vi "Handle Dirty Elements.vi"(8 "Update Time":i32=100, 10 "notifier out":refnum<notifier>, 11 "IsClient":bool) -> (2 "notifier out 2":refnum<notifier>)   [LabVIEW 2017]
doc: "Based on the update rate of this client, keep track of elements that are dirty - have been written to locally. Propagate those values to other clients. This VI also injects statistical measurements of the NT traffic and stores modified value to the persistence file if the variable has been marked as persistent."
uses:
  <vilib>/Rock Robotics/Network Tables/Make Table Operation.ctl
  <vilib>/Rock Robotics/Network Tables/NT Globals.vi
panel:
  in  "Usage Report Period":dbl=0.5
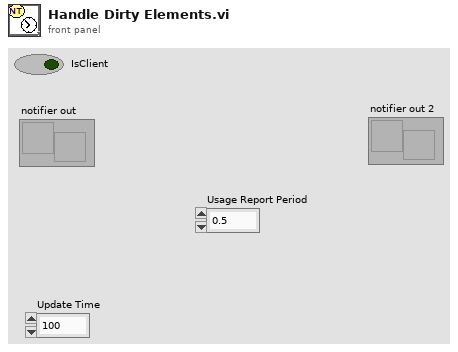
[diagram p1: front panel]
types:
  T1 = enum16{"Add Cnx", "Remove Cnx", "Retrieve List", "Cnx Inited"}
  T2 = typedef "Make Table Operation.ctl" = enum16{"Get or Add Field", "Get Field or Add Temp", "Replace Temp ID", "Get Field ID - No Add", "Get Table Field IDs", "Get Field ID Info", "Move Field to Temp", "Validate", "Remove Field", "Remove All"}
  T3 = typedef "Field ID.ctl" = i32
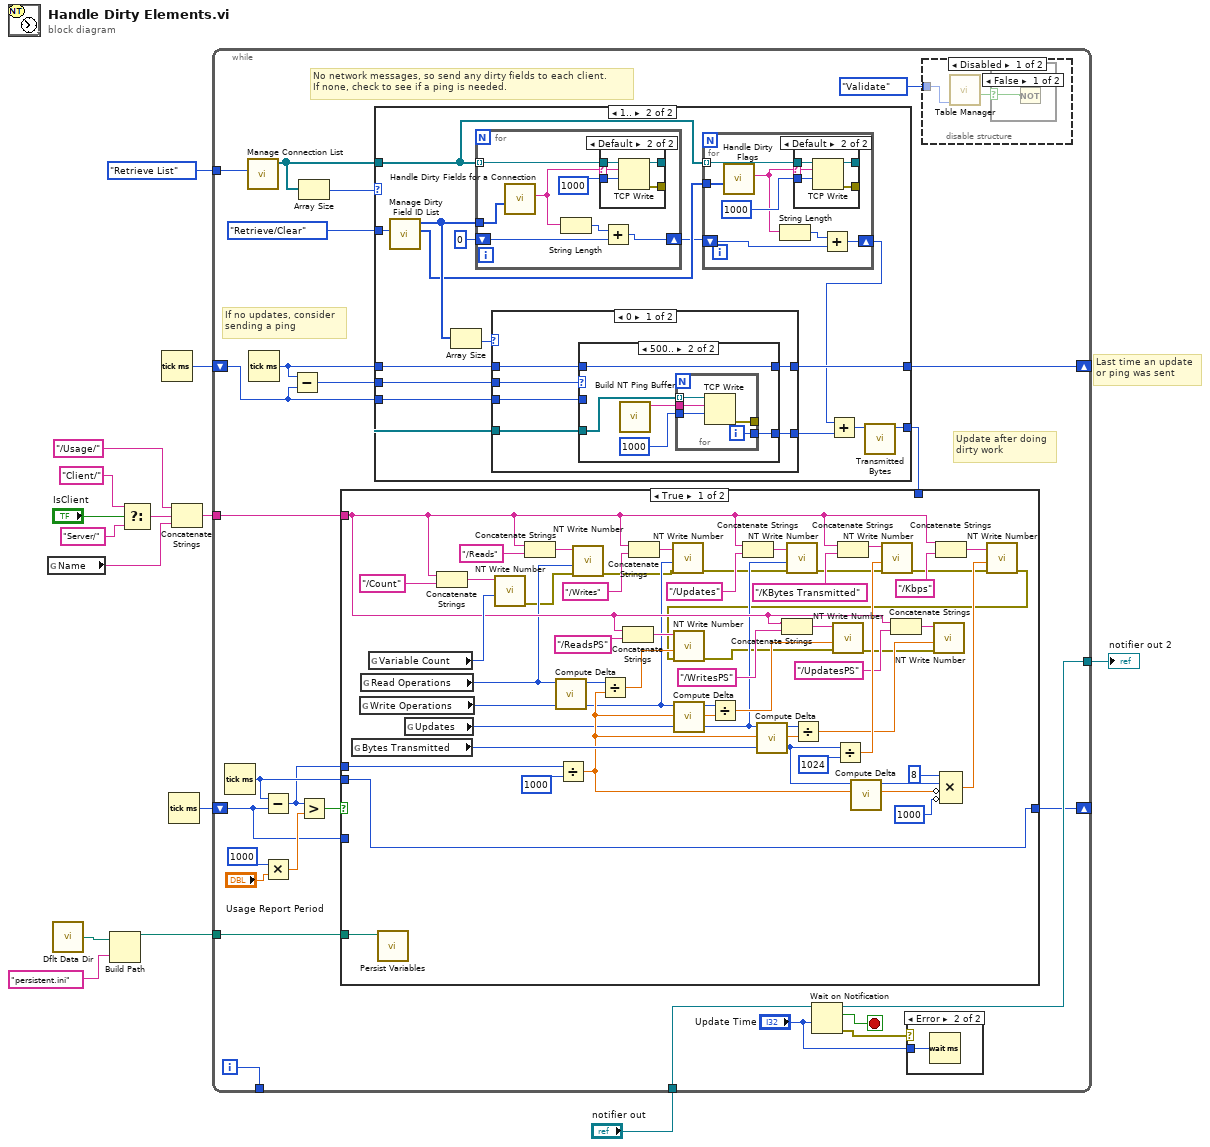
[diagram p0: block diagram]
diagram:
  # "Last time an update\nor ping was sent"
  n1 = global read "NT Globals.vi" "Name"() -> (w12:string)
  n2 = call <vilib>:"Dflt Data Dir.vi"() -> ("App:Default Data Directory"=w1:path)
  n3 = Build Path(base path=w1, name or relative path="persistent.ini") -> (appended path=w2:path)
  n4 = Select(t="Client/" ("Name"), s="IsClient", f="Server/" ("Name")) -> (s? t:f=w11:string)
  n5 = Tick Count (ms)() -> (millisecond timer value=w15:u32)
  n6 = Tick Count (ms)() -> (millisecond timer value=w5:u32)
  n7 = Concatenate Strings("/Usage/" ("Name"), w11, w12) -> (w7:string)
  n8 = while {
    shift-right: [w40] -> _
    shift-left: w15 -> [w34]
    tunnel: "notifier out" -> [w39]
    tunnel: [w38] -> w13
    tunnel: w7 -> [w36]
    tunnel: [w32] -> _
    shift-right: [w26] -> _
    shift-left: w5 -> [w24]
    tunnel: T1."Retrieve List" ("Operation") -> [w17]
    tunnel: w2 -> [w16]
    i -> [w32]
    stop <- w37 stop-if-true
    # "Update after doing\ndirty work"
    # "No network messages, so send any dirty fields to each client.\nIf none, check to see if a ping is needed."
    # "If no updates, consider\nsending a ping"
    n9 = Tick Count (ms)() -> (millisecond timer value=w25:u32)
    n10 = call <vilib>:"Manage Connection List.vi"("Operation"=w17) -> ("Connections List"=w21:refnum<k5>[])  [unwired: 8 in, 2 out]
    n11 = Tick Count (ms)() -> (millisecond timer value=w35:u32)
    n12 = Subtract(x=w25, y=w24) -> (x-y=w23:u32)
    n13 = Multiply(x=1000, y="Usage Report Period") -> (x*y=w27:dbl)
    n14 = Subtract(x=w35, y=w34) -> (x-y=w33:u32)
    n15 = Array Size(array=w21) -> (size(s)=w20:i32)
    n16 = Greater?(x=w23, y=w27) -> (0:w18:bool)
    n17 = case shown="1.." w20 {
      tunnel: enum16{"Mark", "Retrieve/Clear"}."Retrieve/Clear" ("Operation") -> [_ w60]
      tunnel: [w45 w59] -> w40
      tunnel: w35 -> [_ w55]
      tunnel: w34 -> [w45 w54]
      tunnel: w33 -> [_ w53]
      tunnel: w21 -> [_ w48]
      tunnel: [_ w50] -> w19
      frame 0, Default {
      }
      frame 1.. {
        n18 = call <vilib>:"Manage Dirty Field ID List.vi"("Operation"=w60) -> ("Field IDs Flags"=w49:T3[], "Field IDs"=w52:T3[])  [unwired: 9 in]
        n19 = Array Size(array=w52) -> (size(s)=w58:i32)
        n20 = for {
          tunnel: w48 -> [w98] mode=indexing
          tunnel: w52 -> [w97]
          shift-right: [w92] -> w47
          shift-left: 0 -> [w93]
          n21 = call <vilib>:"Handle Dirty Fields for a Connection.vi"("Field IDs"=w97) -> ("String out"=w94:string)  [unwired: 10 in]
          n22 = String Length(string=w94) -> (length=w95:i32)
          n23 = case shown="Default" w94 {
            selector: w94 -> [_ w101]
            tunnel: [_ w104] -> _
            tunnel: [w99 w103] -> _
            tunnel: w98 -> [w99 w102]
            tunnel: 1000 ("timeout ms (25000)") -> [_ w100]
            frame "" {
            }
            frame Default {
              n24 = TCP Write(connection ID=w102, data in=w101, 9:w100) -> (connection ID out=w103:refnum<k5>, error out=w104:errorcluster)  [unwired: 1 in, 1 out]
            }
          }
          n25 = Add(x=w95, y=w93) -> (x+y=w92:i32)
        }
        n26 = case shown="0" w58 {
          tunnel: [w78 w91] -> w59
          tunnel: w55 -> [w79 w91]
          tunnel: w54 -> [w77 _]
          tunnel: w48 -> [w76 _]
          tunnel: [w75 _] -> w57
          tunnel: w53 -> [w74 _]
          frame 0 {
            n27 = case shown="500.." w74 {
              tunnel: w79 -> [_ w85]
              tunnel: [w80 w85] -> w78
              tunnel: w77 -> [w80 _]
              tunnel: w76 -> [_ w83]
              tunnel: [_ w82] -> w75
              frame 0, Default {
              }
              frame 500.. {
                n28 = call <vilib>:"Build NT Ping Buffer.vi"() -> ("Data Buffer"=w84:string)  [unwired: 11 in]
                n29 = for {
                  tunnel: w84 -> [w89]
                  tunnel: w83 -> [w90] mode=indexing
                  tunnel: [w88] -> _
                  tunnel: [w87] -> w82
                  tunnel: 1000 ("timeout ms (25000)") -> [w86]
                  i -> [w87]
                  n30 = TCP Write(connection ID=w90, data in=w89, 9:w86) -> (error out=w88:errorcluster)  [unwired: 1 in, 2 out]
                }
              }
            }
          }
          frame 1, Default {
          }
        }
        n31 = for {
          tunnel: w49 -> [w67]
          tunnel: w48 -> [w65] mode=indexing
          shift-right: [w62] -> w46
          shift-left: w47 -> [w63]
          n32 = call <vilib>:"Handle Dirty Flags.vi"("Field IDs"=w67) -> ("String out"=w61:string)  [unwired: 10 in]
          n33 = String Length(string=w61) -> (length=w64:i32)
          n34 = case shown="Default" w61 {
            selector: w61 -> [_ w70]
            tunnel: [_ w73] -> _
            tunnel: [w68 w72] -> _
            tunnel: w65 -> [w68 w71]
            tunnel: 1000 ("timeout ms (25000)") -> [_ w69]
            frame "" {
            }
            frame Default {
              n35 = TCP Write(connection ID=w71, data in=w70, 9:w69) -> (connection ID out=w72:refnum<k5>, error out=w73:errorcluster)  [unwired: 1 in, 1 out]
            }
          }
          n36 = Add(x=w64, y=w63) -> (x+y=w62:i32)
        }
        n37 = Add(x=w46, y=w57) -> (x+y=w51:i32)
        n38 = call <vilib>:"Transmitted Bytes.vi"("Additional"=w51) -> ("Tally"=w50:i32)  [unwired: 10 in]
      }
    }
    n39 = case shown="True" w18 {
      tunnel: w36 -> [w129 _]
      tunnel: w19 -> [_ _]
      tunnel: w23 -> [w125 _]
      tunnel: [w139 w155] -> w26
      tunnel: w25 -> [w139 _]
      tunnel: w24 -> [_ w155]
      tunnel: w16 -> [w106 _]
      frame True {
        n40 = global read "NT Globals.vi" "Bytes Transmitted"() -> (w138:i32)
        n41 = global read "NT Globals.vi" "Write Operations"() -> (w118:i32)
        n42 = global read "NT Globals.vi" "Read Operations"() -> (w115:i32)
        n43 = global read "NT Globals.vi" "Variable Count"() -> (w152:i32)
        n44 = call <vilib>:"Persist Variables.vi"("Path"=w106) -> ()  [unwired: 11 in]
        n45 = global read "NT Globals.vi" "Updates"() -> (w120:i32)
        n46 = Concatenate Strings(w129, "/Count" ("Name")) -> (w153:string)
        n47 = call <vilib>:"NT Write Number.vi"("Numeric"=w152, "Name"=w153) -> ("error out"=w114:errorcluster)  [unwired: 9 in]
        n48 = Concatenate Strings(w129, "/Reads" ("Name")) -> (w150:string)
        n49 = call <vilib>:"Compute Delta.vi"("value"=w115) -> ("delta"=w116:i32)  [unwired: 10 in]
        n50 = Divide(x=w125, y=1000) -> (x/y=w124:dbl)
        n51 = call <vilib>:"NT Write Number.vi"("error in"=w114, "Numeric"=w115, "Name"=w150) -> ("error out"=w113:errorcluster)  [unwired: 8 in]
        n52 = Divide(x=w116, y=w124) -> (x/y=w133:dbl)
        n53 = Concatenate Strings(w129, "/ReadsPS" ("Name")) -> (w134:string)
        n54 = Concatenate Strings(w129, "/Writes" ("Name")) -> (w148:string)
        n55 = call <vilib>:"NT Write Number.vi"("error in"=w113, "Numeric"=w118, "Name"=w148) -> ("error out"=w112:errorcluster)  [unwired: 8 in]
        n56 = call <vilib>:"Compute Delta.vi"("value"=w118) -> ("delta"=w117:i32)  [unwired: 10 in]
        n57 = Divide(x=w117, y=w124) -> (x/y=w130:dbl)
        n58 = Concatenate Strings(w129, "/Updates" ("Name")) -> (w145:string)
        n59 = call <vilib>:"Compute Delta.vi"("value"=w120) -> ("delta"=w119:i32)  [unwired: 10 in]
        n60 = Concatenate Strings(w129, "/WritesPS" ("Name")) -> (w131:string)
        n61 = call <vilib>:"NT Write Number.vi"("error in"=w112, "Numeric"=w120, "Name"=w145) -> ("error out"=w111:errorcluster)  [unwired: 8 in]
        n62 = Divide(x=w119, y=w124) -> (x/y=w126:dbl)
        n63 = Divide(x=w138, y=1024) -> (x/y=w137:dbl)
        n64 = Concatenate Strings(w129, "/KBytes Transmitted" ("Name")) -> (w144:string)
        n65 = call <vilib>:"Compute Delta.vi"("value"=w138) -> ("delta"=w121:i32)  [unwired: 10 in]
        n66 = call <vilib>:"NT Write Number.vi"("error in"=w111, "Numeric"=w137, "Name"=w144) -> ("error out"=w110:errorcluster)  [unwired: 8 in]
        n67 = Concatenate Strings(w129, "/UpdatesPS" ("Name")) -> (w128:string)
        n68 = Concatenate Strings(w129, "/Kbps" ("Name")) -> (w143:string)
        n69 = Compound Arithmetic op=MULTIPLY(8, w121, invert w124, invert 1000) -> (w141:dbl)
        n70 = call <vilib>:"NT Write Number.vi"("error in"=w110, "Numeric"=w141, "Name"=w143) -> ("error out"=w107:errorcluster)  [unwired: 8 in]
        n71 = call <vilib>:"NT Write Number.vi"("error in"=w107, "Numeric"=w133, "Name"=w134) -> ("error out"=w109:errorcluster)  [unwired: 8 in]
        n72 = call <vilib>:"NT Write Number.vi"("error in"=w109, "Numeric"=w130, "Name"=w131) -> ("error out"=w108:errorcluster)  [unwired: 8 in]
        n73 = call <vilib>:"NT Write Number.vi"("error in"=w108, "Numeric"=w126, "Name"=w128) -> ()  [unwired: 8 in, 1 out]
      }
      frame False {
      }
    }
    n74 = Wait on Notification(notifier=w39, timeout in ms (-1)="Update Time") -> (notifier out=w38:refnum<notifier>, notification=w37:bool, error out=w31:errorcluster)  [unwired: 2 in, 1 out]
    n75 = case shown="Error" w31 {
      tunnel: "Update Time" -> [_ w105]
      frame No Error {
      }
      frame Error {
        n76 = Wait (ms)(milliseconds to wait=w105) -> ()  [unwired: 1 out]
      }
    }
    n77 = disable-structure shown="Disabled" {
      disable-tunnel: Make_Table_Operation."Validate" ("Operation") -> [w43 _]
      frame Disabled {
        n78 = call <vilib>:"Table Manager.vi"("Operation"=w43) -> ("Success"=w42:bool)  [unwired: 7 in, 3 out]
        n79 = case shown="False" w42 {
          selector: w42 -> [w44 _]
          frame False {
            n80 = Not(x=w44) -> ()  [unwired: 1 out]
          }
          frame True {
          }
        }
      }
      frame Enabled {
      }
    }
  }
  "notifier out 2" <- w13
